vi "ContPreProc.vi"(6 "step num":i32, 8 "error in (no error)":errorcluster, 10 "Compiler Settings":T3={"Python Path"=path "", "Main File"="makesequence.py", "Meta File"="makesequence.py", "Aux File"="makesequence.py", "Pre File"="metascript.txt"}, 11 "Enum":enum16{"Meta", "Aux", "Main"}(ring)) -> (0 "error out":errorcluster, 1 "string seq out":string, 3 "Main pulse seq":T1, 5 "calib":bool, 7 "CompileSuccess?":bool=TRUE)   [LabVIEW 2019]
uses:
  PulseCompiler/CompilerSettings.ctl
  PulseControl.ctl
  Compiler/Params.ctl
  Log/GlobalPyConsole.vi
  controls/GlobalExp.vi
  Global.lvlib
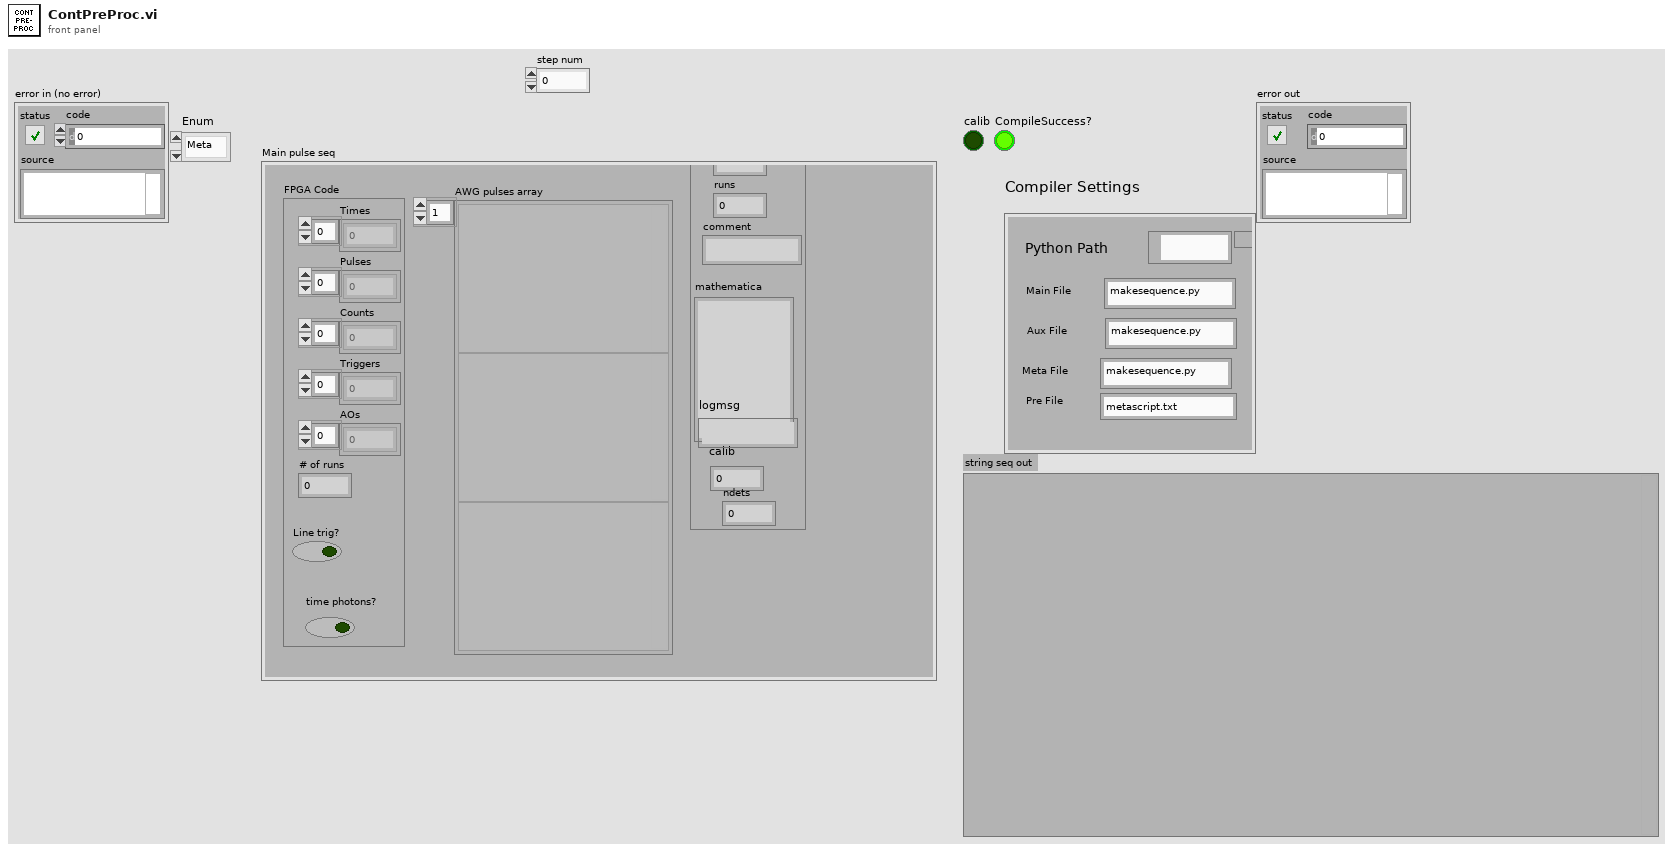
[diagram p1: front panel]
types:
  T1 = typedef "PulseControl.ctl" = cluster{"FPGA Code":cluster{"Times":u32[], "Pulses":u64[], "Counts":u8[], "Triggers":u8[], "AOs":u8[], "# of runs":i32, "Line trig?":bool, "time photons?":bool}, "AWG pulses array":variant[], "Params":T2}
  T2 = typedef "Params.ctl" = cluster{"steps":i16, "runs":i16, "comment":string, "mathematica":string, "calib":i8, "logmsg":string, "ndets":i16}
  T3 = typedef "CompilerSettings.ctl" = cluster{"Python Path":path, "Main File":string, "Meta File":string, "Aux File":string, "Pre File":string}
  T4 = typedef "SinglePulse.ctl" = cluster{"enabled":bool, "string":string, "time":dbl, "step":dbl, "dio":dbl, "count":dbl, "trigger":dbl, "AO":dbl}
  T5 = cluster{u32[], dbl[], "Count":dbl[], dbl[], dbl[], "# of runs":i32, "Line trig":bool, "save photon times":bool}
  T6 = typedef "MasterExpControl.ctl" = cluster{"Main Steps":dbl, "Main Runs":dbl, "ExpStatus":enum16{"Innit", "Stop", "Idle", "MainRunning", "AuxRunning"}, "Main Current Step":dbl, "ExpNum":dbl, "NewData":bool, "date":string, "command":string, "Stop":bool, "Pause":bool, "Mathematica":string, "Main/Meta":bool, "UpdateMath":bool, "Camera":bool, "MetaExpOver":bool, "NextMetaExp":bool}
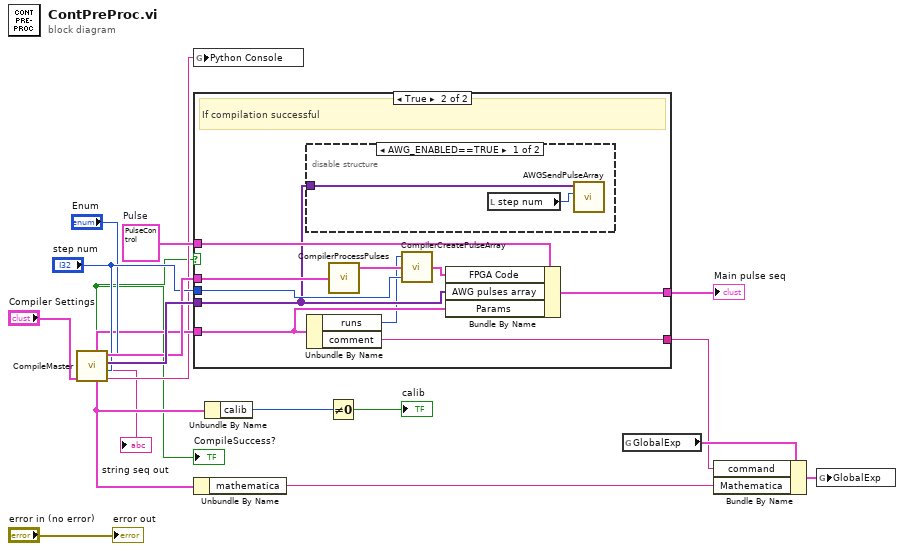
[diagram p0: block diagram]
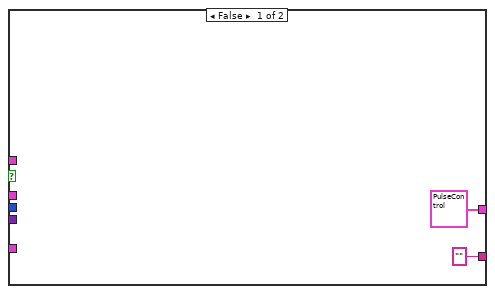
[diagram p2: hidden frame]
diagram:
  w15 = T1 {"FPGA Code"={"Times"=[], "Pulses"=[], "Counts"=[], "Triggers"=[], "AOs"=[], "# of runs"=0, "Line trig?"=FALSE, "time photons?"=FALSE}, "AWG pulses array"=[], "Params"={"steps"=0, "runs"=0, "comment"="", "mathematica"="", "calib"=0, "logmsg"="", "ndets"=0}}  # Pulse
  n1 = call "CompileMaster.vi"("Type"="Enum", "Stepnum"="step num", "Compiler Settings"="Compiler Settings") -> ("CompileSuccess?"=w3:bool, "Params"=w7:T2, "PulseList"=w14:T4[], "RF Array"=w17:variant[], "standard output"=→"string seq out":string, "Standard Error Out"=w4:string)  [unwired: 1 in]
  "CompileSuccess?" <- w3
  n2 = global write "GlobalPyConsole.vi" "Python Console"(w4) -> ()
  n3 = case shown="True" w3 {
    tunnel: w17 -> [_ w24]
    tunnel: [T1 {"FPGA Code"={"Times"=[], "Pulses"=[], "Counts"=[], "Triggers"=[], "AOs"=[], "# of runs"=0, "Line trig?"=FALSE, "time photons?"=FALSE}, "AWG pulses array"=[], "Params"={"steps"=0, "runs"=0, "comment"="", "mathematica"="", "calib"=0, "logmsg"="", "ndets"=0}} ("Pulse") w30] -> w16
    tunnel: w15 -> [_ w29]
    tunnel: w14 -> [_ w28]
    tunnel: "step num" -> [_ w25]
    tunnel: w7 -> [_ w23]
    tunnel: ["" ("comment") w22] -> w2
    frame False {
    }
    frame True {
      # "If compilation successful"
      n4 = disable-structure shown="AWG_ENABLED==TRUE" {
        disable-tunnel: w24 -> [w32 _]
        frame condition #0 (active) {
          n5 = local read "step num"() -> (w31:i32)
          n6 = call "AWGSendPulseArray.vi"("Step Number"=w31, "AWG pulses array"=w32) -> ()  [unwired: 9 in, 1 out]
        }
        frame condition #1 {
        }
      }
      n7 = Unbundle By Name(w23) -> ("runs"=w21:i16, "comment"=w22:string)
      n8 = call "CompilerProcessPulses.vi"("Pulse Seq In"=w28) -> ("Pulse Seq Out"=w27:T4[])  [unwired: 2 out]
      n9 = call "CompilerCreatePulseArray.vi"("step #"=w25, "Pulse Seq In"=w27, "runs"=w21) -> ("Pulse Seq Out"=w26:T5)
      n10 = Bundle By Name(cluster=w29, "FPGA Code"=w26, "AWG pulses array"=w24, "Params"=w23) -> (w30:T1)
    }
  }
  "Main pulse seq" <- w16
  n11 = Unbundle By Name(w7) -> ("mathematica"=w10:string)
  n12 = Unbundle By Name(w7) -> ("calib"=w6:i8)
  n13 = Not Equal To 0?(x=w6) -> (x != 0?=→"calib":bool)
  n14 = global read "GlobalExp.vi" "GlobalExp"() -> (w11:T6)
  n15 = Bundle By Name(cluster=w11, "command"=w2, "Mathematica"=w10) -> (w9:T6)
  n16 = global write "GlobalExp.vi" "GlobalExp"(w9) -> ()
  "error out" <- "error in (no error)"
